vi "Get Oldest File in Directory.vi"(8 "error in":errorcluster, 11 "Directory":path) -> (0 "error out":errorcluster, 3 "Oldest File":path)   [LabVIEW 2027, in "Embedded Data Logger Windows System Tests.lvclass"]
uses:
  Embedded Data Logger Windows System Tests.lvclass
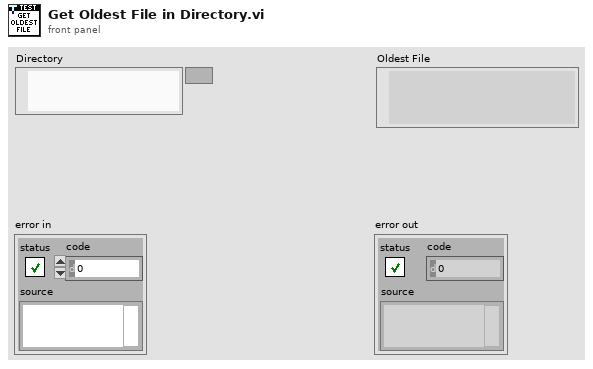
[diagram p1: front panel]
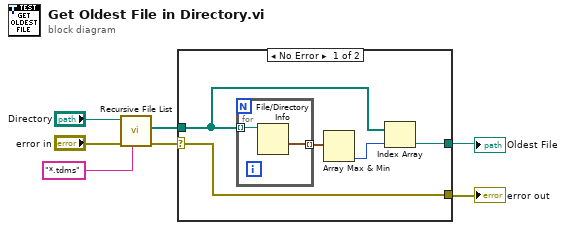
[diagram p0: block diagram]
diagram:
  n1 = call <vilib>:"Recursive File List.vi"("pattern"="*.tdms", "error in (no error)"="error in", "Folder Path"="Directory") -> ("error out"=w1:errorcluster, "All Files in Dir"=w2:path[])  [unwired: 4 in, 3 out]
  n2 = case shown="No Error" w1 {
    selector: w1 -> [w12 w15]
    tunnel: w2 -> [w10 _]
    tunnel: [w12 w15] -> w3
    tunnel: [w8 _] -> w6
    frame No Error {
      n3 = for {
        tunnel: w10 -> [w14] mode=indexing
        tunnel: [w13] -> w11 mode=indexing
        n4 = File/Directory Info(path=w14) -> (last mod=w13:timestamp)  [unwired: 1 in, 6 out]
      }
      n5 = Array Max & Min(array=w11) -> (min index (indices)=w9:i32)  [unwired: 3 out]
      n6 = Index Array(array=w10, index=w9) -> (element=w8:path)
    }
    frame Error {
      # "Error - Most likely source path doesn't exist"
    }
  }
  "Oldest File" <- w6
  "error out" <- w3
